vi "PH_SystemInformation.get Timing Mode.vi"(0 "i ref in":refnum<vi>, 5 "error in (no error)":errorcluster) -> (14 "i ref out":refnum<vi>, 17 "PHELIX Timing Mode":enum32{"10 Hz", "0.5 Hz", "Shot"}(ring), 19 "error out":errorcluster)   [LabVIEW 2014, in "PH_SystemInformation.lvlib"]
doc: "By this VI the current timing mode is requested."
uses:
  PH_SystemInformation.lvlib
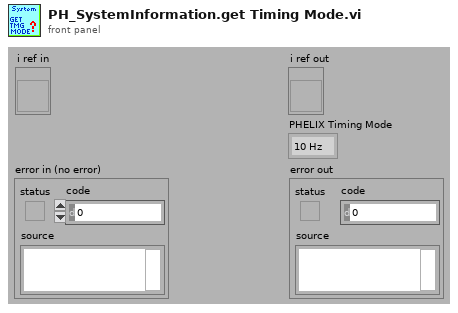
[diagram p1: front panel]
types:
  T1 = typedef "PH_SystemInformation.lvlib/PH_SystemInformation.i attribute.ctl" = cluster{"Laser Enabling":cluster{"GUI Ref":refnum<vi>, "Enabling State":T2}, "PreAmp Enabling":cluster{"GUI Ref":refnum<vi>, "Enabling State":T2}, "MainAmp Enabling":cluster{"GUI Ref":refnum<vi>, "Enabling State":T2}, "Emergency Off":cluster{"GUI Ref":refnum<vi>, "State":enum16{"no info", "off/false", "Alarm"}}, "Enabling Exp. 1":cluster{"GUI Ref":refnum<vi>, "Enabling State":T2}, "Enabling Exp. 2":cluster{"GUI Ref":refnum<vi>, "Enabling State":T2}, "Enabling Exp. 3":cluster{"GUI Ref":refnum<vi>, "Enabling State":T2}, "Enabling Exp. 4":cluster{"GUI Ref":refnum<vi>, "Enabling State":T2}, "Timing Mode":cluster{"GUI Ref":refnum<vi>, "PHELIX_Timing_Mode":enum32{"10 Hz", "0.5 Hz", "Shot"}}}
  T2 = typedef "PH_SystemInformation.lvlib/PH_SystemInformationEnabling State.ctl" = i32
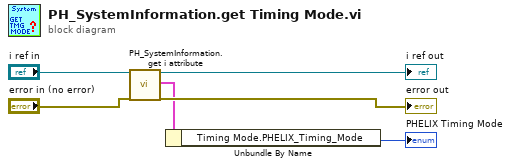
[diagram p0: block diagram]
diagram:
  n1 = call "PH_SystemInformation.get i attribute.vi"("i ref in"="i ref in", "error in (no error)"="error in (no error)") -> ("i ref out"=→"i ref out":refnum<vi>, "i attribute"=w2:T1, "error out"=→"error out":errorcluster)  [unwired: 15 in]
  n2 = Unbundle By Name(w2) -> ("Timing Mode.PHELIX_Timing_Mode"=→"PHELIX Timing Mode":enum32{"10 Hz", "0.5 Hz", "Shot"})
